vi "dfd_Render ZPK Function.vi"(0 "picture in":picture, 1 "fonts input":T2(array[cluster]), 2 "format coeffiecients":string="%#_g", 3 "variable":string="z", 5 "numerator roots":cdb[](array[numeric]), 7 "denominator roots":cdb[](array[numeric]), 9 "gain":dbl, 10 "alignment(left, top)":T1, 11 "rect in":T3, 12 "display format":T4 items=["Separated Roots", "Combined Roots"], 13 "bracket":cluster{"left":string, "right":string}={"left"="(", "right"=")"}, 15 "delay":dbl) -> (4 "picture out":picture, 6 "rect out":T3={"left"=0, "top"=0, "right"=90, "bottom"=34})   [LabVIEW 2017, in "NI_DigFilter_Process.lvlib"]
uses:
  <vilib>/addons/Digital Filter Design/NI_DigFilter_Process.lvlib
  <vilib>/addons/Digital Filter Design/Render.llb/dfd_ZPK Display Format.ctl
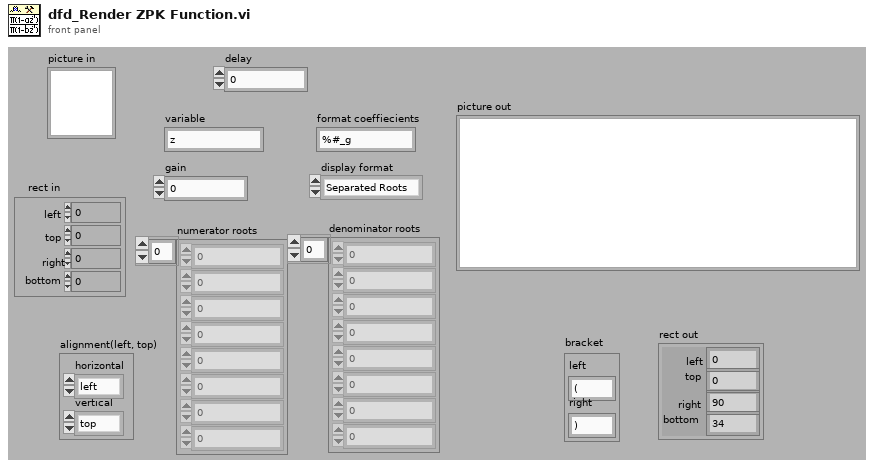
[diagram p1: front panel]
types:
  T1 = cluster{"horizontal":enum16{"left", "center", "right"}, "vertical":enum16{"top", "center", "bottom"}}
  T2 = cluster{"Font Name:":string, "Size":i16, "Strikeout?":bool, "Italic?":bool, "Underline?":bool, "Outline?":bool, "Shadow?":bool, "Bold?":bool}[]
  T3 = cluster{"left":i16, "top":i16, "right":i16, "bottom":i16}
  T4 = typedef "dfd_ZPK Display Format.ctl" = u16
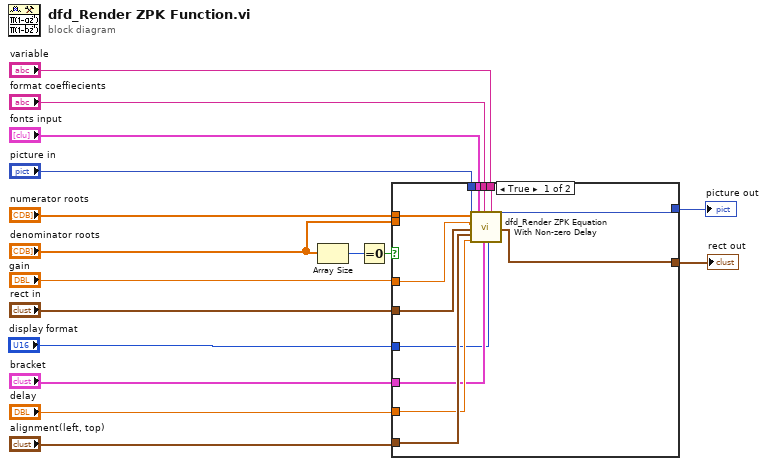
[diagram p0: block diagram]
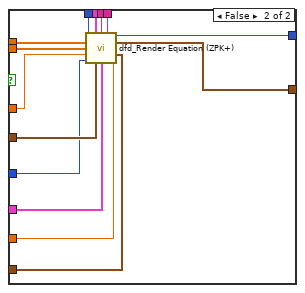
[diagram p2: hidden frame]
diagram:
  n1 = Array Size(array="denominator roots") -> (size(s)=w3:i32)
  n2 = Equal To 0?(x=w3) -> (x = 0?=w2:bool)
  n3 = case shown="True" w2 {
    tunnel: "numerator roots" -> [w24 w43]
    tunnel: "fonts input" -> [w28 w42]
    tunnel: "format coeffiecients" -> [w27 w41]
    tunnel: "variable" -> [w26 w40]
    tunnel: "gain" -> [w23 w39]
    tunnel: "rect in" -> [w17 w38]
    tunnel: "delay" -> [w21 w37]
    tunnel: [w29 w36] -> w8
    tunnel: "display format" -> [w18 w30]
    tunnel: [w19 w35] -> w6
    tunnel: "alignment(left, top)" -> [w22 w34]
    tunnel: "bracket" -> [w20 w33]
    tunnel: "picture in" -> [w25 w32]
    tunnel: "denominator roots" -> [_ w31]
    frame True {
      n4 = call <vilib>:"dfd_Render ZPK Equation With Non-zero Delay.vi"("picture in"=w25, "roots"=w24, "gain"=w23, "rect in"=w17, "alignment(left, top)"=w22, "delay"=w21, "Fonts Input"=w28, "format coeffiecients"=w27, "bracket"=w20, "variable"=w26, "display format"=w18) -> ("picture out"=w29:picture, "total rect"=w19:T3)  [unwired: 7 out]
    }
    frame False {
      n5 = call <vilib>:"dfd_Render Equation (ZPK+).vi"("picture in"=w32, "fonts input"=w42, "format coeffiecients"=w41, "variable"=w40, "numerator roots"=w43, "denominator roots"=w31, "gain"=w39, "alignment(left, top)"=w34, "display format"=w30, "rect in"=w38, "bracket"=w33, "delay"=w37) -> ("picture out"=w36:picture, "rect out"=w35:T3)  [unwired: 1 in, 1 out]
    }
  }
  "picture out" <- w8
  "rect out" <- w6
